vi "Obtain-DAQ-Queue.vi"() -> (6 "DAQ-Queue":refnum<queue>)   [LabVIEW 2014, in "HISW.lvclass"]
doc: "Obtain a queue for DAQ acquisition\nany of the three Qtypes (PAQ/WAQ/EAQ) can write to this HISW Queue"
uses:
  HISW.lvclass
  controls/typedef-DAQ-datagram.ctl
  controls/typedef-Qtype.ctl
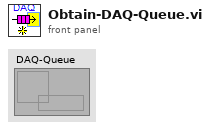
[diagram p1: front panel]
types:
  T1 = typedef "typedef-DAQ-datagram.ctl" = cluster{"Time Stamp":timestamp, "Source":string, "Data":variant, "Qtype":T2}
  T2 = typedef "typedef-Qtype.ctl" = enum16{"PAQ", "WAQ", "EAQ", "End-Service"}
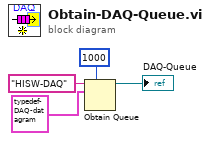
[diagram p0: block diagram]
diagram:
  n1 = Obtain Queue(max queue size (-1, unlimited)=1000, name (unnamed)="HISW-DAQ", element data type=T1 {"Time Stamp"=timestamp(0 s since 1904-01-01), "Source"="", "Data"=variant, "Qtype"=enum."PAQ"} ("DAQ-datagram")) -> (queue out=→"DAQ-Queue":refnum<queue>)  [unwired: 2 in, 2 out]
